vi "Johnson_lindenstrauss_min_dim.vi"(8 "error in":errorcluster caption="entrée d'erreur", 11 "johnson_lindenstrauss_min_dim":cluster{"n_samples":i32[], "eps":dbl[]} {"eps" min=0.0 max=1.0}) -> (0 "error out":errorcluster caption="sortie d'erreur", 3 "Data":T1)   [LabVIEW 2020]
doc: "Find a ‘safe’ number of components to randomly project to\n\nThe distortion introduced by a random projection p only changes the distance between two points by a factor (1 +- eps) in an euclidean space with good probability. The projection p is an eps-embedding as defined by:\n\n(1 - eps) ||u - v||^2 < ||p(u) - p(v)||^2 < (1 + eps) ||u - v||^2\n\nWhere u and v are any rows taken from a dataset of shape [n_samples, n_features], eps is in ]0, 1[ and p is a projection by a random Gaussian N(0, 1) matrix with shape [n_components, n_features] (or a sparse Achlioptas matrix).\n\nThe minimum number of components to guarantee the eps-embedding is given by:\n\nn_components >= 4 log(n_samples) / (eps^2 / 2 - eps^3 / 3)\n\nNote that the number of dimensions is independent of the original number of features but instead depends on the size of the dataset: the larger the dataset, the higher is the minimal dimensionality of an eps-embedding.\n\n\nParameters :\n\n- n_samples : int or numpy array of int greater than 0,\nNumber of samples. If an array is given, it will compute a safe number of components array-wise.\n\n- eps : float or numpy array of float in ]0,1[, optional (default=0.1)\nMaximum distortion rate as defined by the Johnson-Lindenstrauss lemma. If an array is given, it will compute a safe number of components array-wise.\n\nReturns :\n\n- n_components : int or numpy array of int,\nThe minimal number of components to guarantee with good probability an eps-embedding with n_samples."
uses:
  Johnson_lindenstrauss_min_dim.lvclass
panel:
  out "Johnson_lindenstrauss_min_dim.lvclass":refnum<class "Johnson_lindenstrauss_min_dim.lvclass">
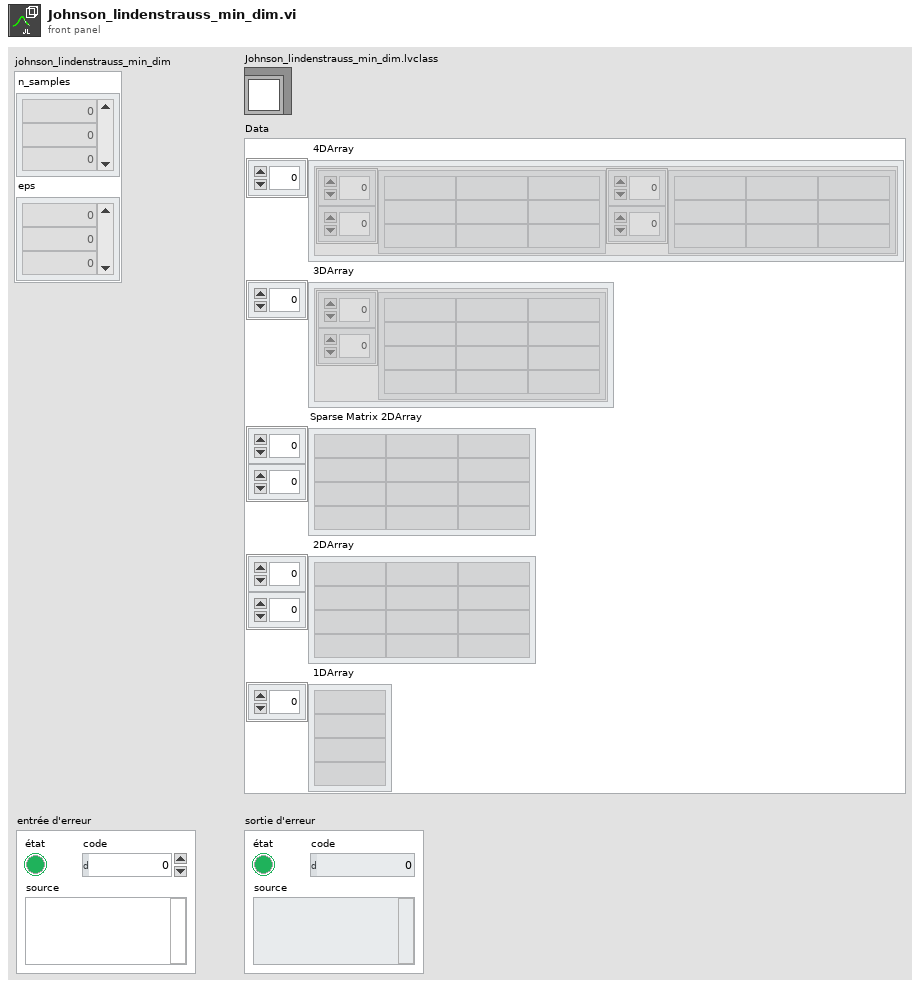
[diagram p1: front panel]
types:
  T1 = cluster{" 4DArray":cluster{"1":string[][], "2":string[][]}[], " 3DArray":cluster{"Tableau":string[][]}[], "Sparse Matrix 2DArray":string[][], " 2DArray":string[][], " 1DArray":string[]}
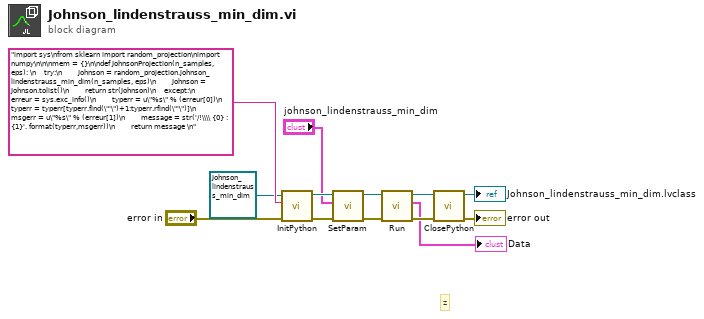
[diagram p0: block diagram]
diagram:
  # "z"
  n1 = call-dynamic "InitPython.vi"("error in (no error)"="error in", "Python Instruction"="import sys\nfrom sklearn import random_projection\nimport numpy\n\n\nmem = {}\n\ndef JohnsonProjection(n_samples, eps): \n    try:\n        Johnson = random_projection.johnson_lindenstrauss_min_dim(n_samples, eps)\n        Johnson = Johnson.tolist()\n        return str(Johnson)\n    except:\n        erreur = sys.exc_info()\n        typerr = u\"%s\" % (erreur[0])\n        typerr = typerr[typerr.find(\"'\")+1:typerr.rfind(\"'\")]\n        msgerr = u\"%s\" % (erreur[1])\n        message = str('/!\\\\ {0} : {1}'. format(typerr,msgerr))\n        return message \n", "Scikit-learn en entrée"=refnum<class "Johnson_lindenstrauss_min_dim.lvclass"> refnum ("Johnson_lindenstrauss_min_dim.lvclass")) -> ("error out"=w9:errorcluster, "Scikit-learn en sortie"=w10:refnum<class "Johnson_lindenstrauss_min_dim.lvclass">)  [unwired: 7 in]
  n2 = call-dynamic "SetParam.vi"("error in (no error)"=w9, "johnson_lindenstrauss_min_dim"="johnson_lindenstrauss_min_dim", "Johnson_lindenstrauss_min_dim.lvclass"=w10) -> ("error out"=w7:errorcluster, "Johnson_lindenstrauss_min_dim.lvclass"=w8:refnum<class "Johnson_lindenstrauss_min_dim.lvclass">)  [unwired: 7 in]
  n3 = call-dynamic "Run.vi"("error in (no error)"=w7, "Johnson_lindenstrauss_min_dim.lvclass"=w8) -> ("error out"=w5:errorcluster, "Data"=→"Data":T1, "Johnson_lindenstrauss_min_dim.lvclass"=w4:refnum<class "Johnson_lindenstrauss_min_dim.lvclass">)  [unwired: 7 in]
  n4 = call-dynamic "ClosePython.vi"("error in (no error)"=w5, "Scikit-learn en entrée"=w4) -> ("error out"=→"error out":errorcluster, "Scikit-learn en sortie"=→"Johnson_lindenstrauss_min_dim.lvclass":refnum<class "Johnson_lindenstrauss_min_dim.lvclass">)  [unwired: 8 in]
